vi "CodeDetection2(SubVI).vi"(2 "Code":dbl[](array[numeric]), 3 "Buff":dbl[][](array[numeric]), 4 "L_sum":i32) -> (0 "detect":bool, 1 "Position":dbl[](array[numeric]))   [LabVIEW 2017]
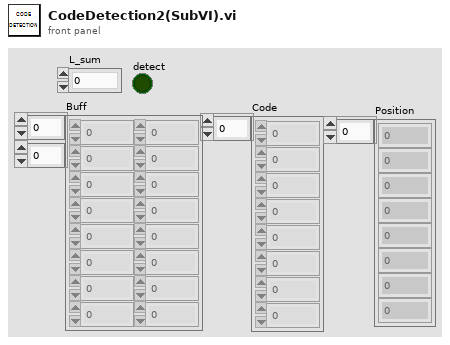
[diagram p1: front panel]
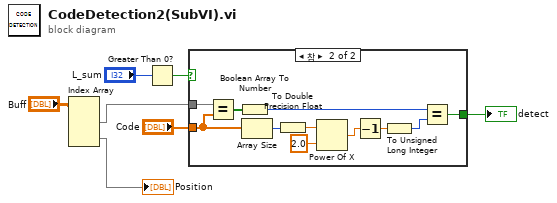
[diagram p0: block diagram]
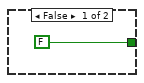
[diagram p2: hidden frame]
diagram:
  n1 = Index Array(array="Buff") -> (element #1=w2:dbl[], element #2=→"Position":dbl[])  [unwired: 4 in]
  n2 = Greater Than 0?(x="L_sum") -> (x > 0?=w6:bool)
  n3 = case shown="참" w6 {
    tunnel: [FALSE w14] -> w4
    tunnel: "Code" -> [_ w16]
    tunnel: w2 -> [_ w17]
    frame False {
    }
    frame True {
      n4 = Equal?(x=w17, y=w16) -> (x = y?=w19:bool[])
      n5 = Boolean Array To Number(Boolean array=w19) -> (number=w18:u32)
      n6 = Array Size(array=w16) -> (size(s)=w12:i32)
      n7 = To Double Precision Float(number=w12) -> (double precision float=w11:dbl)
      n8 = Power Of X(1:2.0 ("x"), 2:w11) -> (0:w10:dbl)
      n9 = Decrement(x=w10) -> (x-1=w15:dbl)
      n10 = To Unsigned Long Integer(number=w15) -> (unsigned 32bit integer=w9:u32)
      n11 = Equal?(x=w18, y=w9) -> (x = y?=w14:bool)
    }
  }
  "detect" <- w4
